vi "Update Subscription Arrays on Unsubscribe.vi"(9 "UnSubscribe Topic Array":string[](array[string]), 10 "ViewerRef in":T1[](array[typedef]), 11 "subscriptionList in":string[](array[string])) -> (1 "ViewerRef's to close":T1[](array[typedef]), 2 "ViewerRef out":T1[](array[typedef]), 3 "subscriptionList out":string[](array[string]))   [LabVIEW 2018]
uses:
  viewer/controls/viewewr_bus.ctl
  viewer/TopicViewer.lvlib
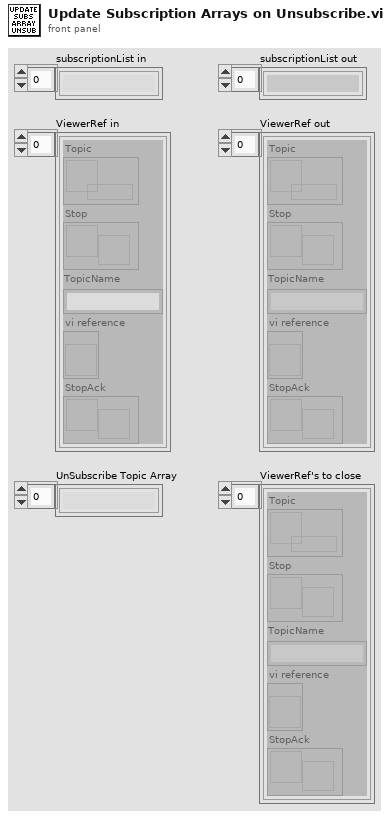
[diagram p1: front panel]
types:
  T1 = typedef "TopicViewer.lvlib/viewewr_bus.ctl" = cluster{"Topic":refnum<queue>, "Stop":refnum<notifier>, "TopicName":string, "vi reference":refnum<vi>, "StopAck":refnum<notifier>}
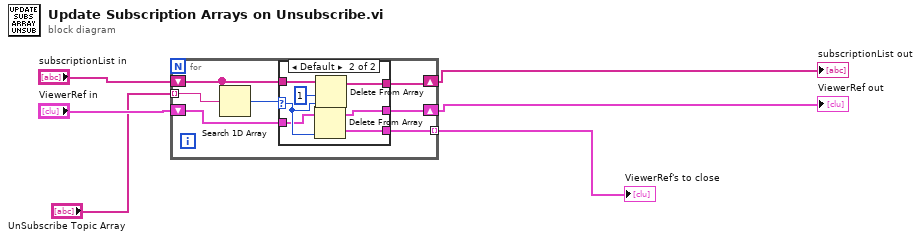
[diagram p0: block diagram]
diagram:
  n1 = for {
    shift-right: [w10] -> w3
    shift-left: "subscriptionList in" -> [w11]
    tunnel: "UnSubscribe Topic Array" -> [w13] mode=indexing
    shift-right: [w8] -> w5
    shift-left: "ViewerRef in" -> [w9]
    tunnel: [w7] -> w6 mode=indexing
    n2 = Search 1D Array(1D array=w11, element=w13) -> (index of element=w12:i32)  [unwired: 1 in]
    n3 = case shown="Default" w12 {
      selector: w12 -> [_ w19]
      tunnel: w11 -> [w15 w22]
      tunnel: [w15 w21] -> w10
      tunnel: w9 -> [w14 w18]
      tunnel: [w14 w17] -> w8
      tunnel: [_ w16] -> w7
      frame -1 {
      }
      frame Default {
        n4 = Delete From Array(array=w18, index=w19) -> (deleted portion=w16:T1, array with subset deleted=w17:T1[])  [unwired: 1 in]
        n5 = Delete From Array(array=w22, length=1, index=w19) -> (array with subset deleted=w21:string[])  [unwired: 1 out]
      }
    }
  }
  "ViewerRef's to close" <- w6
  "ViewerRef out" <- w5
  "subscriptionList out" <- w3
